vi "Get_File_info.vi"() -> ()   [LabVIEW 2011]
panel:
  out "error out":errorcluster
  in  "file path":path
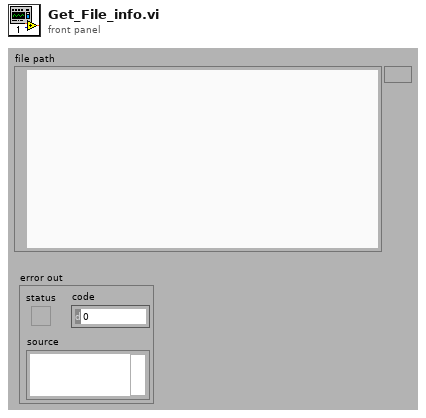
[diagram p1: front panel]
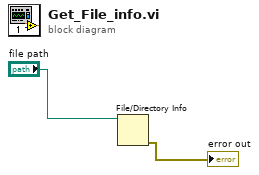
[diagram p0: block diagram]
diagram:
  n1 = File/Directory Info(path="file path") -> (error out=→"error out":errorcluster)  [unwired: 1 in, 6 out]
